vi "Write Enabled.vi"(8 "error in (no error)":errorcluster, 10 "Enabled?":bool[](array[boolean]), 11 "Change Laser Frequency in":refnum<class "Change Laser Enable State.lvclass">) -> (0 "error out":errorcluster, 3 "Change Laser Frequency out":refnum<class "Change Laser Enable State.lvclass">)   [LabVIEW 2014, in "ePAS Library.lvlib" / "Change Laser Enable State.lvclass"]
uses:
  Change Laser Enable State.lvclass
  Change Laser Enable State.lvclass/Change Laser Enable State.ctl
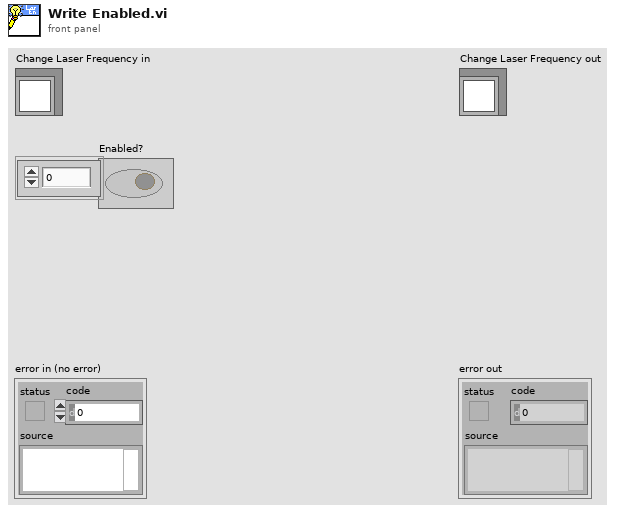
[diagram p1: front panel]
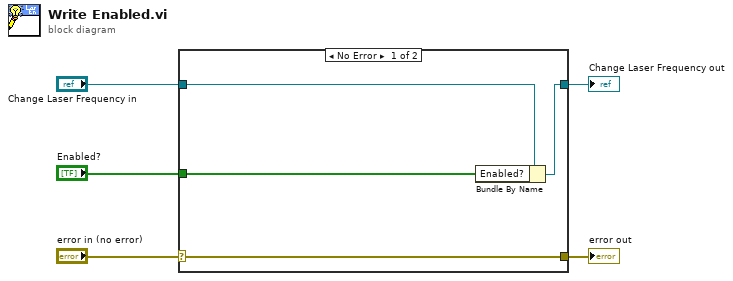
[diagram p0: block diagram]
diagram:
  n1 = case shown="No Error" "error in (no error)" {
    selector: "error in (no error)" -> [w9 w10]
    tunnel: [w9 w10] -> w4
    tunnel: [w7 w11] -> w2
    tunnel: "Change Laser Frequency in" -> [w8 w11]
    tunnel: "Enabled?" -> [w6 _]
    frame No Error {
      n2 = Bundle By Name(cluster=w8, "Enabled?"=w6) -> (w7:refnum<class "Change Laser Enable State.lvclass">)
    }
    frame Error {
    }
  }
  "error out" <- w4
  "Change Laser Frequency out" <- w2
